vi "main_ctrl.vi"(8 "error in":errorcluster) -> (0 "error out":errorcluster caption="error")   [LabVIEW 2013]
uses:
  <vilib>/Rock Robotics/WPI/DriverStation/WPI_DriverStationRobotMode2.ctl
  typedefs/fg_typedef.ctl
  typedefs/vision enable.ctl
  typedefs/vision data.ctl
  typedefs/subStates.ctl
  typedefs/singleUseSubstate.ctl
  <vilib>/Rock Robotics/WPI/Solenoid/WPI_SolenoidValue.ctl
  <vilib>/Rock Robotics/WPI/RobotDrive/WPI_RobotDriveGetSetRefNum.vi
  <vilib>/Rock Robotics/WPI/RobotDrive/WPI_RobotDriveArcadeDrive_Standard(NoSaturation).vi
  <vilib>/Rock Robotics/WPI/Solenoid/WPI_SolenoidSetEnum.vi
  <vilib>/Rock Robotics/WPI/Compressor/WPI_CompressorGetSetRefNum.vi
panel:
  out "Enabled?":bool
  out "Robot Mode":T1
  out "Vision SPI":u32
  out "Vision IPS":dbl
  out "Main IPS":dbl
  out "Main SPI":u32
  # "MAIN CONTROL"
  # "holds robot control code - dual parallel state machine"
  # "SPI: milliseconds per iteration\nIPS: iterations per second"
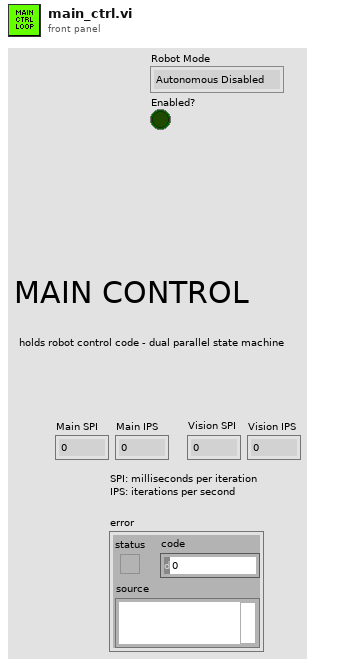
[diagram p1: front panel]
types:
  T1 = typedef "WPI_DriverStationRobotMode2.ctl" = enum16{"Autonomous Disabled", "Autonomous Enabled", "Teleop Disabled", "Teleop Enabled", "Timeout", "Finish", "Test Disabled", "Test Enabled"}
  T2 = typedef "vision data.ctl" = cluster{"x":dbl, "y":dbl, "area":dbl, "width":dbl, "height":dbl, "Hot Goal Present?":bool, "distance":dbl}
  T3 = typedef "vision enable.ctl" = enum16{"Enable", "Disable", "Stop"}
  T4 = typedef "fg_typedef.ctl" = enum16{"Get", "Set"}
  T5 = typedef "WPI_RobotDriveDevRef.ctl" = cluster{"DevStatus":errorcluster, "Motors[]":T6[], "Square Inputs":bool, "Max Output":dbl, "Isochronous":bool}
  T6 = typedef "WPI_MotorControlDeviceRef.ctl" = cluster{"DeviceStatus":errorcluster, "Type":enum16{"PWM", "CAN"}, "PWM":cluster{"Digital Module":T7, "PWM Channel":T8, "DeadBand":T9}, "CAN":cluster{"Device Number":u8, "Control Mode":T10, "Semaphore":T11, "Max Vout":dbl}, "Invert":bool, "TransformRef":T12, "InvTransformRef":T12}
  T7 = typedef "FPGA_TypedefDigitalModule.ctl" = enum16{"Digital Module 1", "Digital Module 2"}
  T8 = typedef "FPGA_DIOPWMChannel.ctl" = enum8{"PWM 1", "PWM 2", "PWM 3", "PWM 4", "PWM 5", "PWM 6", "PWM 7", "PWM 8", "PWM 9", "PWM 10", "Invalid"}
  T9 = typedef "WPI_PWMDeadband.ctl" = cluster{"Name":string, "maxPositivePwm":i32, "minPositivePwm":i32, "centerPwm":i32, "maxNegativePwm":i32, "minNegativePwm":i32, "angularRange":u16}
  T10 = typedef "WPI_CANJaguar_ControlMode.ctl" = enum8{"Percent VBus", "Current", "Speed", "Position", "Voltage"}
  T11 = typedef "Semaphore RefNum" = refnum<k1>
  T12 = typedef "WPI_PWMTransform_ConPane.ctl" = refnum<vi>
  T13 = typedef "WPI_SolenoidDevRef.ctl" = cluster{"DevStatus":errorcluster, "Solenoid Module":T14, "Forward Solenoid Channel":T15, "Reverse Solenoid Channel":T15}
  T14 = typedef "FPGA_TypedefSolenoidModule.ctl" = enum16{"Solenoid Module 1", "Solenoid Module 2"}
  T15 = typedef "WPI_SolenoidChannel.ctl" = enum8{"Solenoid 1", "Solenoid 2", "Solenoid 3", "Solenoid 4", "Solenoid 5", "Solenoid 6", "Solenoid 7", "Solenoid 8", "Invalid"}
  T16 = typedef "WPI_CameraDevRef.ctl" = cluster{"Camera Address":string, "CameraStatus":errorcluster, "Acquire Image Notifier":refnum<notifier>}
  T17 = typedef "WPI_CompressorDevRef.ctl" = cluster{"DevStatus":errorcluster, "DigitalInputDevRef":T18, "RelayDevRef":T20}
  T18 = typedef "WPI_DigitalInputDevRef.ctl" = cluster{"DevStatus":errorcluster, "DIO Channel":T19, "Digital Module":T7}
  T19 = typedef "FPGA_DIOChannel.ctl" = enum8{"DIO 1", "DIO 2", "DIO 3", "DIO 4", "DIO 5", "DIO 6", "DIO 7", "DIO 8", "DIO 9", "DIO 10", "DIO 11", "DIO 12", "DIO 13", "DIO 14", "Invalid"}
  T20 = typedef "WPI_RelayDevRef.ctl" = cluster{"DevStatus":errorcluster, "Relay Channel":T21, "Digital Module":T7, "Relay Direction":T22}
  T21 = typedef "FPGA_DIORelayChannel.ctl" = enum8{"Relay 1", "Relay 2", "Relay 3", "Relay 4", "Relay 5", "Relay 6", "Relay 7", "Relay 8", "Invalid"}
  T22 = typedef "WPI_RelayDirection.ctl" = enum16{"Both directions", "Forward only", "Reverse only"}
  T23 = typedef "IMAQ Image.ctl" = refnum<image>
  T24 = typedef "WPI_SolenoidValue.ctl" = enum16{"Off", "On", "Forward", "Reverse"}
  T25 = typedef "singleUseSubstate.ctl" = enum16{"null", "wait", "shift high", "shift low"}
  T26 = typedef "subStates.ctl" = enum16{"null", "wait", "driver control", "auto", "manual override", "hold position", "rotate", "pickup", "pass", "load", "goto shoot", "shoot", "end"}
  T27 = typedef "WPI_DriverStationDerivedRobotMode.ctl" = enum16{"Init", "Execute", "Stop"}
  T28 = typedef "Loop 0 Datatype.ctl" = cluster{"State":T26, "Waiting Loop":i32, "State to Wait For":i32, "Loop ID":i32, "Exit Value":i32, "X Axis":dbl, "Y Axis":dbl, "Z Axis":dbl}
  T29 = cluster{"Vision mSPI":u32, "Main mSPI":u32, "Dash mSPI":u32}
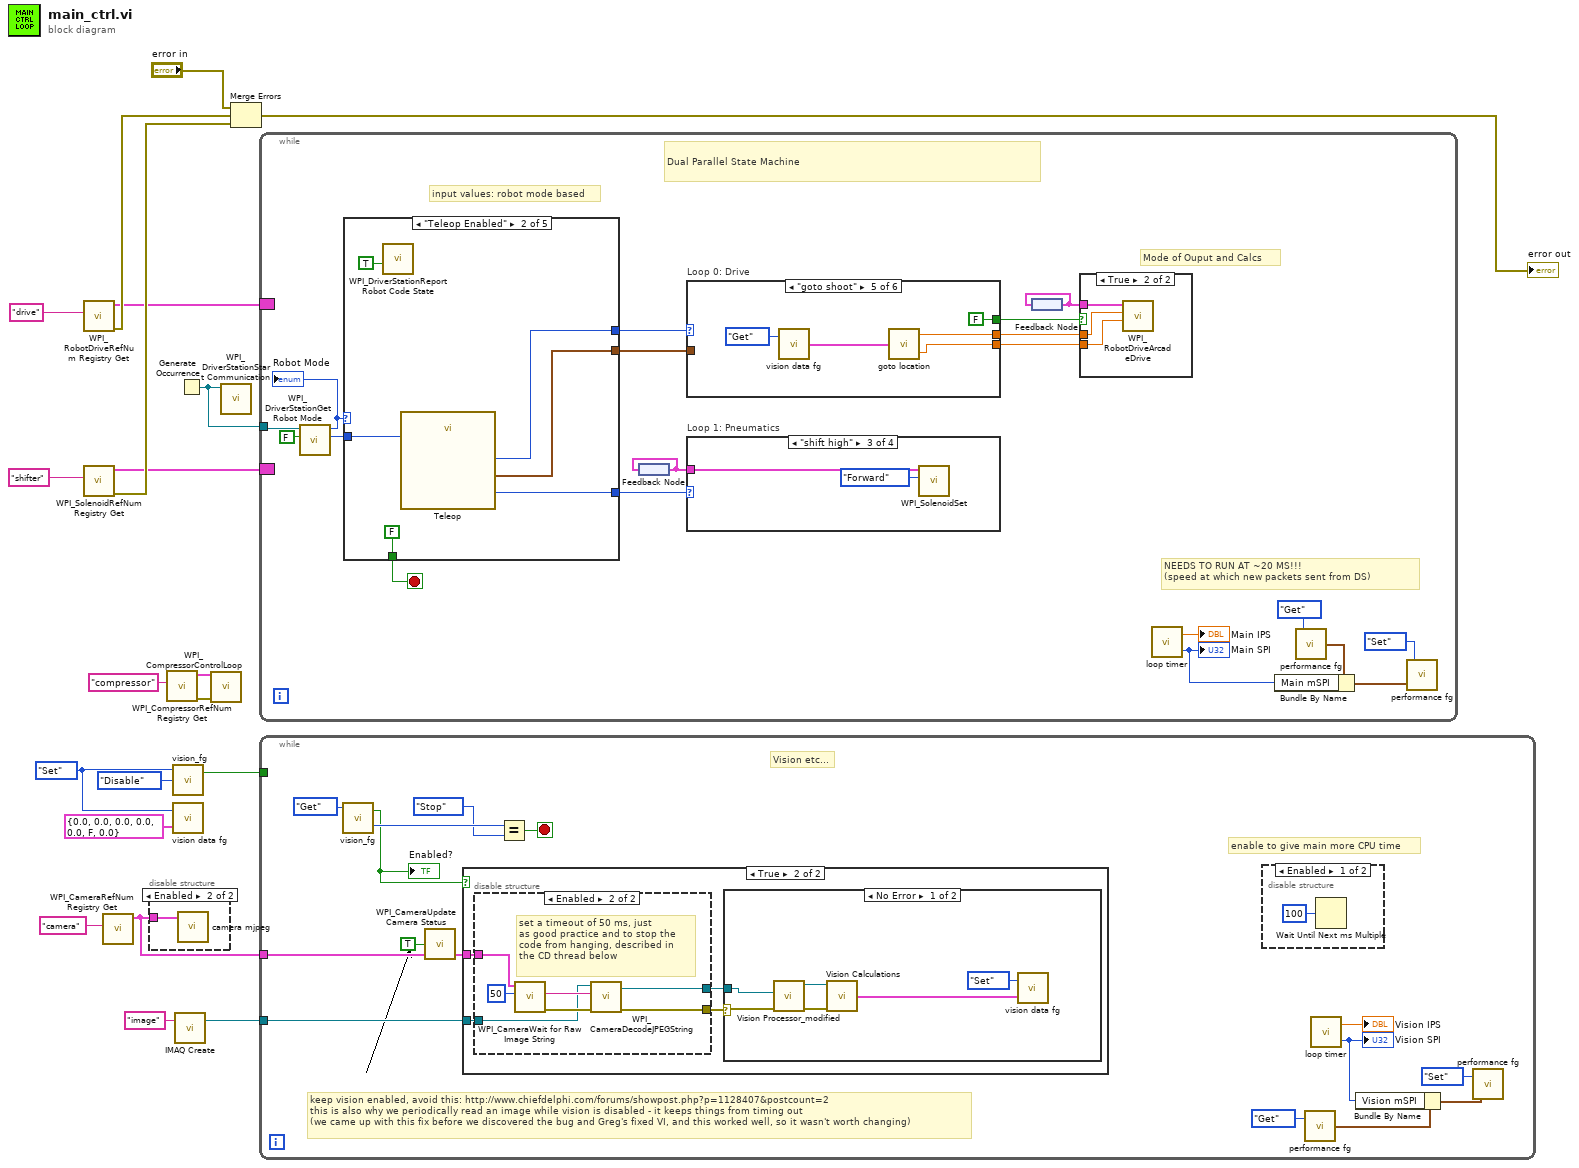
[diagram p0: block diagram]
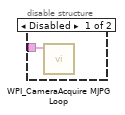
[diagram p2: hidden frame]
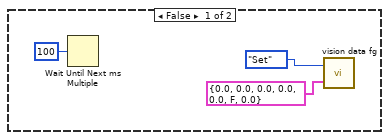
[diagram p4: hidden frame]
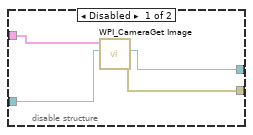
[diagram p6: hidden frame]
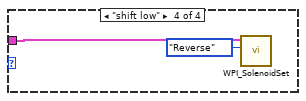
[diagram p9: hidden frame]
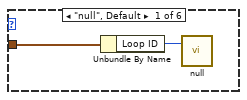
[diagram p10: hidden frame]
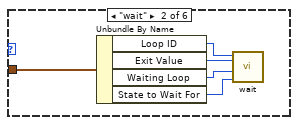
[diagram p11: hidden frame]
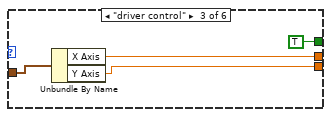
[diagram p12: hidden frame]
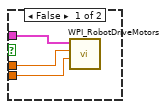
[diagram p15: hidden frame]
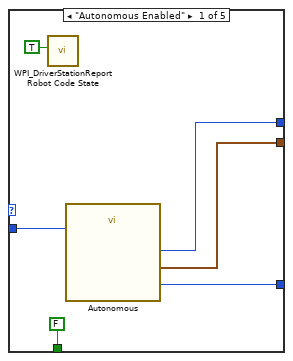
[diagram p16: hidden frame]
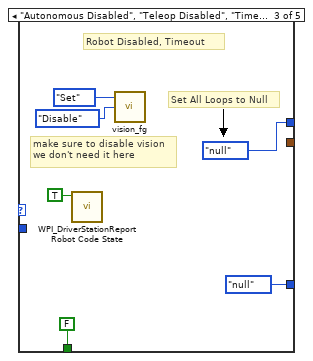
[diagram p17: hidden frame]
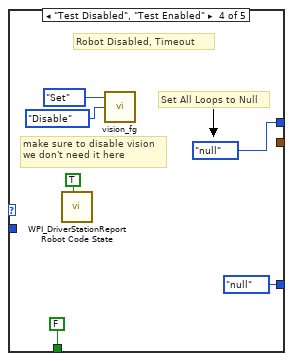
[diagram p18: hidden frame]
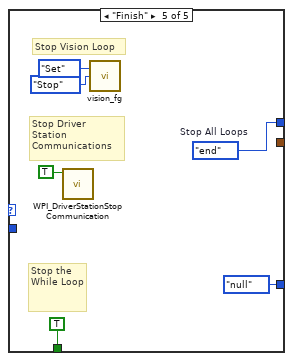
[diagram p19: hidden frame]
diagram:
  w12 = fg_typedef."Set" ("Enum")
  n1 = call <vilib>:"WPI_RobotDriveRefNum Registry Get.vi"("refnum name"="drive") -> ("error out"=w7:errorcluster, "RobotDriveDevRef"=w5:T5)  [unwired: 9 in]
  n2 = call <vilib>:"WPI_SolenoidRefNum Registry Get.vi"("refnum name"="shifter") -> ("error out"=w6:errorcluster, "SolenoidDevRef"=w3:T13)  [unwired: 9 in]
  n3 = call <vilib>:"WPI_CameraRefNum Registry Get.vi"("refnum name"="camera") -> ("CameraDevRef"=w9:T16)  [unwired: 9 in, 1 out]
  n4 = disable-structure shown="Enabled" {
    disable-tunnel: w9 -> [w21 w22]
    frame Disabled {
      n5 = call <vilib>:"WPI_CameraAcquire MJPG Loop.vi"("CameraDevRef"=w21) -> ()  [unwired: 11 in]
    }
    frame Enabled {
      n6 = call "camera mjpeg.vi"("CameraDevRef"=w22) -> ()  [unwired: 11 in]
    }
  }
  n7 = call <vilib>:"WPI_CompressorRefNum Registry Get.vi"("refnum name"="compressor") -> ("error out"=w17:errorcluster, "CompressorDevRef"=w16:T17)  [unwired: 9 in]
  n8 = call "vision_fg.vi"("Action"=vision_enable."Disable", "Menu"=w12) -> ("Enabled?"=w13:bool)  [unwired: 1 in, 1 out]
  n9 = call "vision data fg.vi"("Input"=T2 {"x"=0.0, "y"=0.0, "area"=0.0, "width"=0.0, "height"=0.0, "Hot Goal Present?"=FALSE, "distance"=0.0}, "Menu"=w12) -> ()  [unwired: 1 out]
  n10 = call "IMAQ Create"("Image Name"="image") -> ("New Image"=w14:T23)  [unwired: 4 in, 1 out]
  n11 = Generate Occurrence() -> (w20:refnum<k4>)
  n12 = call <vilib>:"WPI_CompressorControlLoop.vi"("error in (no error)"=w17, "CompressorDevRef"=w16) -> ()  [unwired: 10 in]
  n13 = call <vilib>:"WPI_DriverStationStart Communication.vi"("occurrence"=w20) -> ()  [unwired: 11 out]
  n14 = Merge Errors("error in", w7, w6) -> (→"error out":errorcluster)
  n15 = while {
    tunnel: w20 -> [w30]
    border: w5 -> [_]
    border: w3 -> [_]
    stop <- w39 stop-if-true
    # "input values: robot mode based"
    # "Mode of Ouput and Calcs"
    # "NEEDS TO RUN AT ~20 MS!!!\n(speed at which new packets sent from DS)"
    # "Dual Parallel State Machine"
    n16 = call <vilib>:"WPI_DriverStationGet Robot Mode.vi"("Finish"=FALSE, "DS Occurrence"=w30) -> ("Call Context"=w28:T27, "Robot Mode"=w29:T1)  [unwired: 8 out]
    "Robot Mode" <- w29
    n17 = case shown="\"Teleop Enabled\"" w29 {
      tunnel: w28 -> [w68 w76 _ _ _]
      tunnel: [w69 w78 singleUseSubstate."null" ("SubState 5") singleUseSubstate."null" ("SubState 5") singleUseSubstate."null" ("SubState 5")] -> w40
      tunnel: [FALSE FALSE FALSE FALSE TRUE] -> w39
      tunnel: [w71 w75 subStates."null" ("SubState 0") subStates."null" ("SubState 0") w92] -> w32
      tunnel: [w70 w74 _ _ _] -> w33
      frame "Autonomous Enabled" {
        n18 = call <vilib>:"WPI_DriverStationReport Robot Code State.vi"("Autonomous"=TRUE) -> ()  [unwired: 10 in, 1 out]
        n19 = call "Autonomous.vi"("Call Context"=w68) -> ("SubState 0"=w71:T26, "Loop 0 Data"=w70:T28, "SubState 1"=w69:T25)  [unwired: 8 in]
      }
      frame "Teleop Enabled" {
        n20 = call <vilib>:"WPI_DriverStationReport Robot Code State.vi"("TeleOp"=TRUE) -> ()  [unwired: 10 in, 1 out]
        n21 = call "Teleop.vi"("Call Context"=w76) -> ("SubState 1"=w78:T25, "SubState 0"=w75:T26, "Loop 0 Data"=w74:T28)  [unwired: 16 in]
      }
      frame "Autonomous Disabled", "Teleop Disabled", "Timeout" {
        # "Set All Loops to Null"
        # "make sure to disable vision\nwe don't need it here"
        # "Robot Disabled, Timeout"
        n22 = call <vilib>:"WPI_DriverStationReport Robot Code State.vi"("Disabled"=TRUE) -> ()  [unwired: 10 in, 1 out]
        n23 = call "vision_fg.vi"("Action"=vision_enable."Disable", "Menu"=fg_typedef."Set") -> ()  [unwired: 1 in, 2 out]
      }
      frame "Test Disabled", "Test Enabled" {
        # "Set All Loops to Null"
        # "make sure to disable vision\nwe don't need it here"
        # "Robot Disabled, Timeout"
        n24 = call <vilib>:"WPI_DriverStationReport Robot Code State.vi"("Test"=TRUE) -> ()  [unwired: 10 in, 1 out]
        n25 = call "vision_fg.vi"("Action"=vision_enable."Disable", "Menu"=fg_typedef."Set") -> ()  [unwired: 1 in, 2 out]
      }
      frame "Finish" {
        w92 = subStates."end"  # Stop All Loops
        # "Stop the While Loop"
        # "Stop Driver Station Communications"
        # "Stop Vision Loop"
        n26 = call <vilib>:"WPI_DriverStationStop Communication.vi"("StopCommunication"=TRUE) -> ()  [unwired: 10 in, 1 out]
        n27 = call "vision_fg.vi"("Action"=vision_enable."Stop", "Menu"=fg_typedef."Set") -> ()  [unwired: 1 in, 2 out]
      }
    }
    n28 = feedback #1() -> (w23:T13)
    n29 = feedback-in #1(w23) -> ()
    n30 = case "Loop 0: Drive" shown="\"goto shoot\"" w32 {
      tunnel: w33 -> [w46 w48 w56 _ _ _]
      tunnel: [_ _ w55 _ w60 _] -> w27
      tunnel: [_ _ w54 _ w61 _] -> w26
      tunnel: [_ _ TRUE _ FALSE _] -> w25
      frame "null", Default {
        n31 = Unbundle By Name(w46) -> ("Loop ID"=w47:i32)
        n32 = call "null.vi"("This Loop ID"=w47) -> ()  [unwired: 2 in]
      }
      frame "wait" {
        n33 = Unbundle By Name(w48) -> ("Loop ID"=w52:i32, "Exit Value"=w51:i32, "Waiting Loop"=w50:i32, "State to Wait For"=w49:i32)
        n34 = call "wait.vi"("State to wait for"=w49, "Waiting Loop ID"=w50, "time (ms)"=w51, "Current Loop ID"=w52) -> ()  [unwired: 1 out]
      }
      frame "driver control" {
        n35 = Unbundle By Name(w56) -> ("X Axis"=w55:dbl, "Y Axis"=w54:dbl)
      }
      frame "hold position" {
      }
      frame "goto shoot" {
        n36 = call "vision data fg.vi"("Menu"=fg_typedef."Get") -> ("Output"=w58:T2)  [unwired: 1 in]
        n37 = call "goto location.vi"("Image Data"=w58) -> ("left speed"=w60:dbl, "right speed"=w61:dbl)
      }
      frame "manual override" {
      }
    }
    n38 = case "Loop 1: Pneumatics" shown="\"shift high\"" w40 {
      tunnel: w23 -> [_ _ w43 w44]
      frame "null", Default {
      }
      frame "wait" {
      }
      frame "shift high" {
        n39 = call-poly <vilib>:"WPI_SolenoidSet.vi"("Value"=WPI_SolenoidValue."Forward", "SolenoidDevRef"=w43) -> ()  [unwired: 8 in, 2 out]
      }
      frame "shift low" {
        n40 = call-poly <vilib>:"WPI_SolenoidSet.vi"("Value"=WPI_SolenoidValue."Reverse", "SolenoidDevRef"=w44) -> ()  [unwired: 8 in, 2 out]
      }
    }
    n41 = feedback #2() -> (w24:T5)
    n42 = feedback-in #2(w24) -> ()
    n43 = case shown="True" w25 {
      tunnel: w24 -> [w62 w67]
      tunnel: w27 -> [w63 w66]
      tunnel: w26 -> [w64 w65]
      frame False {
        n44 = call <vilib>:"WPI_RobotDriveMotors.vi"("RightSpeed"=w64, "LeftSpeed"=w63, "RobotDriveDevRef"=w62) -> ()  [unwired: 6 in, 3 out]
      }
      frame True {
        n45 = call-poly <vilib>:"WPI_RobotDriveArcadeDrive.vi"("Y axis value"=w65, "X axis value"=w66, "RobotDriveDevRef"=w67) -> ()  [unwired: 6 in, 3 out]
      }
    }
    n46 = call "loop timer.vi"() -> ("IPS"=→"Main IPS":dbl, "SPI"=w38:u32)  [unwired: 1 in]
    "Main SPI" <- w38
    n47 = call "performance fg.vi"("Menu"=fg_typedef."Get") -> ("Output"=w35:T29)  [unwired: 1 in]
    n48 = Bundle By Name(cluster=w35, "Main mSPI"=w38) -> (w34:T29)
    n49 = call "performance fg.vi"("Input"=w34, "Menu"=fg_typedef."Set") -> ()  [unwired: 1 out]
  }
  n50 = while {
    tunnel: w14 -> [w111]
    tunnel: w9 -> [w110]
    tunnel: w13 -> [_]
    stop <- w112 stop-if-true
    # "keep vision enabled, avoid this: http://www.chiefdelphi.com/forums/showpost.php?p=1128407&postcount=2\nthis is also why we periodically read an image while vision is disabled - it keeps things from timing out\n(we came up with this fix before we discovered the bug and Greg's fixed VI, and this worked well, so it wasn't worth changing)"
    # "enable to give main more CPU time"
    # "Vision etc..."
    n51 = call "vision_fg.vi"("Menu"=fg_typedef."Get" ("Enum")) -> ("State Out"=w106:T3, "Enabled?"=w98:bool)  [unwired: 2 in]
    "Enabled?" <- w98
    n52 = call <vilib>:"WPI_CameraUpdate Camera Status.vi"("CameraDevRef In"=w110, "Enable Vision"=TRUE) -> ("CameraDevRef Out"=w109:T16)  [unwired: 3 in]
    n53 = case shown="True" w98 {
      tunnel: w111 -> [_ w120]
      tunnel: w109 -> [_ w119]
      frame False {
        n54 = Wait Until Next ms Multiple(millisecond multiple=u32 100) -> ()  [unwired: 1 out]
        n55 = call "vision data fg.vi"("Input"=T2 {"x"=0.0, "y"=0.0, "area"=0.0, "width"=0.0, "height"=0.0, "Hot Goal Present?"=FALSE, "distance"=0.0}, "Menu"=fg_typedef."Set" ("Enum")) -> ()  [unwired: 1 out]
      }
      frame True {
        n56 = disable-structure shown="Enabled" {
          disable-tunnel: w120 -> [w129 w133]
          disable-tunnel: w119 -> [w130 w135]
          disable-tunnel: [w128 w132] -> w118
          disable-tunnel: [w127 w131] -> w117
          frame Disabled {
            n57 = call <vilib>:"WPI_CameraGet Image.vi"("Image"=w129, "CameraDevRef"=w130) -> ("error out"=w127:errorcluster, "Image Out"=w128:T23)  [unwired: 7 in, 1 out]
          }
          frame Enabled {
            # "set a timeout of 50 ms, just\nas good practice and to stop the \ncode from hanging, described in \nthe CD thread below"
            n58 = call <vilib>:"WPI_CameraWait for Raw Image String.vi"("Timeout in ms (-1)"=50, "CameraDevRef"=w135) -> ("error out"=w137:errorcluster, "String"=w136:string)  [unwired: 3 in, 5 out]
            n59 = call <vilib>:"WPI_CameraDecodeJPEGString.vi"("error in"=w137, "Compressed Image"=w136, "Image In"=w133) -> ("error out"=w131:errorcluster, "Image Out"=w132:T23)  [unwired: 3 out]
          }
        }
        n60 = case shown="No Error" w117 {
          selector: w117 -> [w124 _]
          tunnel: w118 -> [w125 _]
          frame No Error {
            n61 = call "Vision Processor_modified.vi"("error in"=w124, "Image In"=w125) -> ("error out"=w122:errorcluster, "Image Out"=w123:T23)  [unwired: 5 in]
            n62 = call "Vision Calculations.vi"("Image In"=w123, "error in"=w122) -> ("Vision Data"=w121:T2)  [unwired: 3 in]
            n63 = call "vision data fg.vi"("Input"=w121, "Menu"=fg_typedef."Set" ("Enum")) -> ()  [unwired: 1 out]
          }
          frame Error {
          }
        }
      }
    }
    n64 = Equal?(x=w106, y=vision_enable."Stop") -> (x = y?=w112:bool)
    n65 = disable-structure shown="Enabled" {
      frame Enabled {
        n66 = Wait Until Next ms Multiple(millisecond multiple=u32 100) -> ()  [unwired: 1 out]
      }
      frame Disabled {
      }
    }
    n67 = call "performance fg.vi"("Menu"=fg_typedef."Get") -> ("Output"=w102:T29)  [unwired: 1 in]
    n68 = call "loop timer.vi"() -> ("IPS"=→"Vision IPS":dbl, "SPI"=w104:u32)  [unwired: 1 in]
    "Vision SPI" <- w104
    n69 = Bundle By Name(cluster=w102, "Vision mSPI"=w104) -> (w101:T29)
    n70 = call "performance fg.vi"("Input"=w101, "Menu"=fg_typedef."Set") -> ()  [unwired: 1 out]
  }
